vi "DownloadSpriteImages.vi"(8 "error in (no error)":errorcluster, 10 "RT_Game.lvlib:Game.lvclass":refnum<class "Game.lvclass">, 11 "SpriteHandler in":refnum<class "SpriteHandler.lvclass">) -> (0 "error out":errorcluster, 2 "RT_Game.lvlib:Game.lvclass 2":refnum<class "Game.lvclass">, 3 "SpriteHandler out":refnum<class "SpriteHandler.lvclass">)   [LabVIEW 2019, in "RT_Game.lvlib" / "SpriteHandler.lvclass"]
uses:
  SpriteHandler.lvclass
  Game/Game.lvclass
  Game/Game.lvclass/Game.ctl
  SpriteHandler.lvclass/SpriteHandler.ctl
  RT_Sprite/RT_Sprite.lvclass/RT_Sprite.ctl
  RT_Sprite/Read Picture.vi
  Game/Read FPGA_ref.vi
  Game/Write FPGA_ref.vi
  <vilib>/rvi/interface/common/niFpgaWaitOnOcc.vi
  <vilib>/Utility/error.llb/Error Cluster From Error Code.vi
  <vilib>/rvi/errors/niLvFpgaAdjustHostInterfaceError.vi
  FPGA_Interface.ctl
  <vilib>/rvi/interface/nirviMethod/nirviMethod.xnode
  FPGA Bitfiles/myriogameconsole_FPGATarget_Main_ntsPRcBZGxk.lvbitx
  RT_Sprite/RT_Sprite.lvclass
  <vilib>/FPGAPlugInAG/myRIO-1900/niLvFpga_WriteFifo_myRIO-1900.vi
  <vilib>/rvi/errors/niLvFpgaMergeErrorWithErrorCode.vi
  <vilib>/FPGAPlugInAG/myRIO-1900/niLvFpga_ConfigureFifo_myRIO-1900.vi
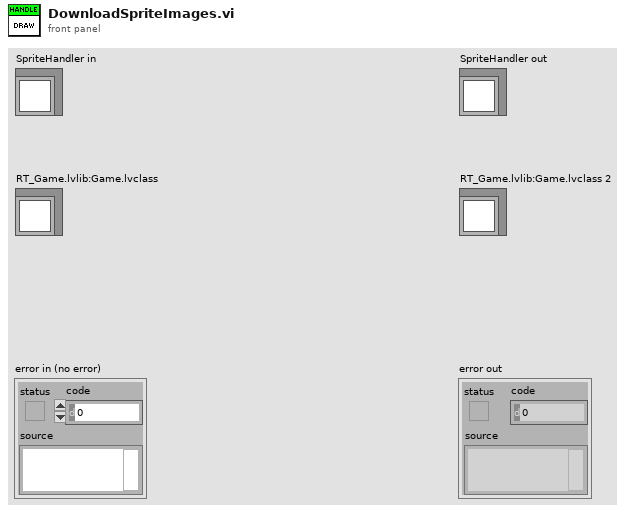
[diagram p1: front panel]
types:
  T1 = typedef "FPGA_Interface.ctl" = refnum<k20>
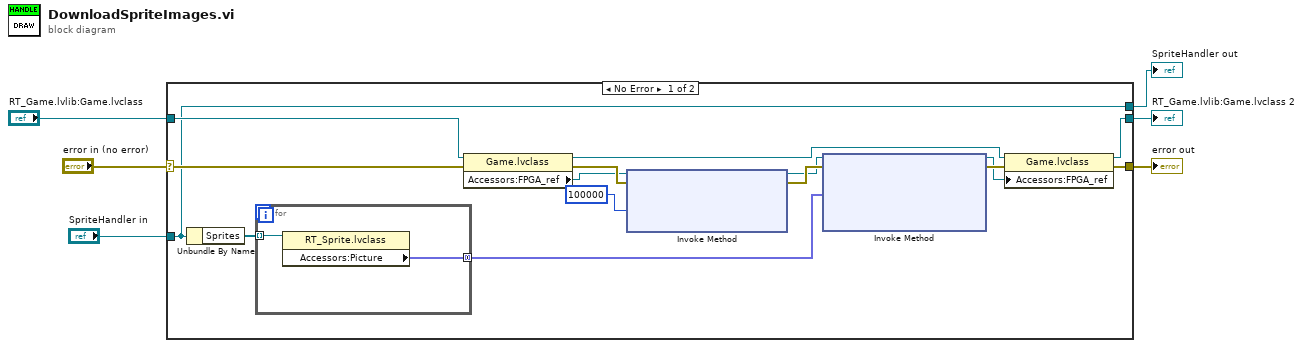
[diagram p0: block diagram]
diagram:
  n1 = case shown="No Error" "error in (no error)" {
    selector: "error in (no error)" -> [w16 w26]
    tunnel: [w17 w26] -> w5
    tunnel: [w13 w25] -> w3
    tunnel: "SpriteHandler in" -> [w13 w25]
    tunnel: [w20 w24] -> w2
    tunnel: "RT_Game.lvlib:Game.lvclass" -> [w21 w24]
    frame No Error {
      n2 = Unbundle By Name(w13) -> ("Sprites"=w12:refnum<class "RT_Sprite.lvclass">[])
      n3 = for {
        tunnel: w12 -> [w23] mode=indexing
        tunnel: [w22] -> w11 mode=concatenating
        n4 = property class="RT_Sprite.lvclass"(reference=w23) -> ("Accessors:Picture"=w22:fxp<+,3,3>[])  [unwired: 1 in, 2 out]
      }
      n5 = property class="Game.lvclass"(reference=w21, error in=w16) -> (reference out=w19:refnum<class "Game.lvclass">, error out=w18:errorcluster, "Accessors:FPGA_ref"=w9:T1)
      n6 = xnode "Invoke Method"("FPGA VI Reference In"=w9, "error in"=w18, "Requested Depth"=u32 100000) -> ("FPGA VI Reference Out"=w8:T1, "error out"=w10:errorcluster)  [unwired: 1 out]
      n7 = xnode "Invoke Method"("FPGA VI Reference In"=w8, "error in"=w10, "Data"=w11) -> ("FPGA VI Reference Out"=w14:T1, "error out"=w15:errorcluster)  [unwired: 1 in, 1 out]
      n8 = property class="Game.lvclass"(reference=w19, error in=w15, "Accessors:FPGA_ref"=w14) -> (reference out=w20:refnum<class "Game.lvclass">, error out=w17:errorcluster)
    }
    frame Error {
    }
  }
  "error out" <- w5
  "SpriteHandler out" <- w3
  "RT_Game.lvlib:Game.lvclass 2" <- w2
